vi "Configure Operational Mode.vi"(8 "error in (no error)":errorcluster, 10 "Operational Mode":u32(ring) items=["Rotary", "Keypad", "Ext Pgm", "Remote"], 11 "VISA resource name":refnum<visa-resource-name>) -> (0 "error out":errorcluster, 3 "VISA resource name out":refnum<visa-resource-name>)   [LabVIEW 2022 SP3, in "MagnaDC.lvlib"]
uses:
  MagnaDC.lvlib
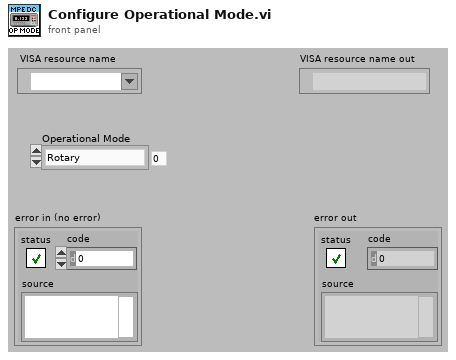
[diagram p1: front panel]
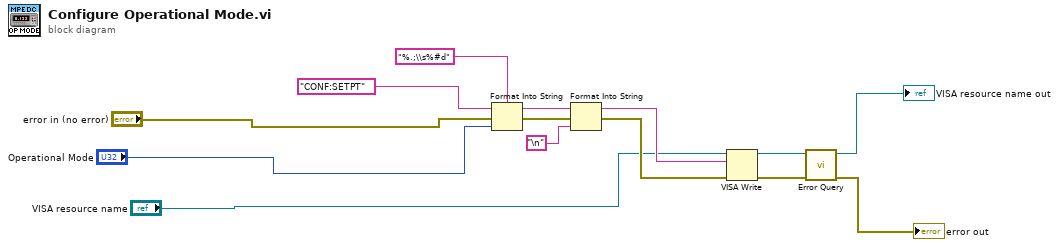
[diagram p0: block diagram]
diagram:
  n1 = Format Into String(format string="%.;\\s%#d", initial string="CONF:SETPT" ("format string"), error in="error in (no error)", "Operational Mode") -> (resulting string=w6:string, error out=w7:errorcluster)
  n2 = Format Into String(initial string=w6, error in=w7, "\n") -> (resulting string=w10:string, error out=w12:errorcluster)  [unwired: 1 in]
  n3 = VISA Write(VISA resource name="VISA resource name", write buffer=w10, error in (no error)=w12) -> (VISA resource name out=w14:refnum<visa-resource-name>, error out=w13:errorcluster)  [unwired: 1 out]
  n4 = call "Error Query.vi"("error in (no error)"=w13, "VISA resource name"=w14) -> ("error out"=→"error out":errorcluster, "VISA resource name out"=→"VISA resource name out":refnum<visa-resource-name>)  [unwired: 6 in, 2 out]
